vi "Get Name.vi"(8 "error in (no error)":errorcluster, 11 "EPU452 in":refnum<class "EPU452.lvclass">) -> (0 "error out":errorcluster, 1 "Name":string, 2 "Response":string, 3 "EPU452 out":refnum<class "EPU452.lvclass">)   [LabVIEW 2018, in "EPU452.lvclass"]
uses:
  EPU452.lvclass
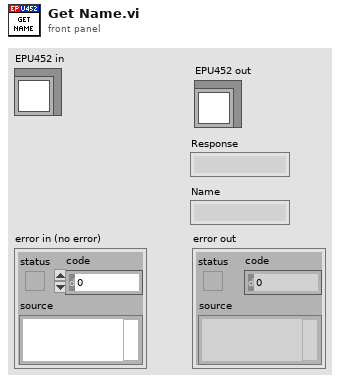
[diagram p1: front panel]
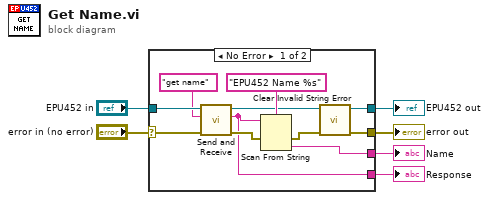
[diagram p0: block diagram]
diagram:
  n1 = case shown="No Error" "error in (no error)" {
    selector: "error in (no error)" -> [w15 w19]
    tunnel: [w8 w19] -> w5
    tunnel: [w7 w18] -> w3
    tunnel: "EPU452 in" -> [w17 w18]
    tunnel: [w10 _] -> w2
    tunnel: [w9 _] -> w1
    frame No Error {
      n2 = call "Send and Receive.vi"("error in (no error)"=w15, "Command"="get name", "EPU452 in"=w17) -> ("error out"=w13:errorcluster, "Response"=w10:string, "EPU452 out"=w11:refnum<class "EPU452.lvclass">)  [unwired: 6 in]
      n3 = Scan From String(format string="EPU452 Name %s", input string=w10, error in=w13) -> (error out=w12:errorcluster, output 1=w9:string)  [unwired: 2 in, 2 out]
      n4 = call "Clear Invalid String Error.vi"("error in (no error)"=w12, "EPU452 in"=w11) -> ("error out"=w8:errorcluster, "EPU452 out"=w7:refnum<class "EPU452.lvclass">)  [unwired: 8 in]
    }
    frame Error {
    }
  }
  "error out" <- w5
  "EPU452 out" <- w3
  "Response" <- w2
  "Name" <- w1
